vi "ex_getNextGroupTDMS.vi"(8 "error in (no error)":errorcluster, 9 "group index in":u32, 11 "tdms file in":refnum<k34>) -> (0 "error out":errorcluster, 1 "group index out":u32, 2 "group name":string, 3 "tdms file out":refnum<k34>, 4 "is last group?":bool, 5 "max len":i32)   [LabVIEW 2017]
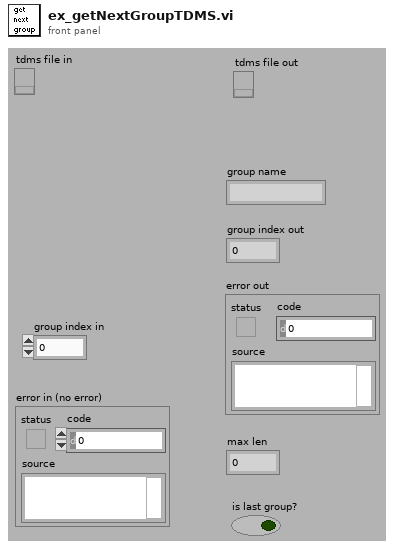
[diagram p1: front panel]
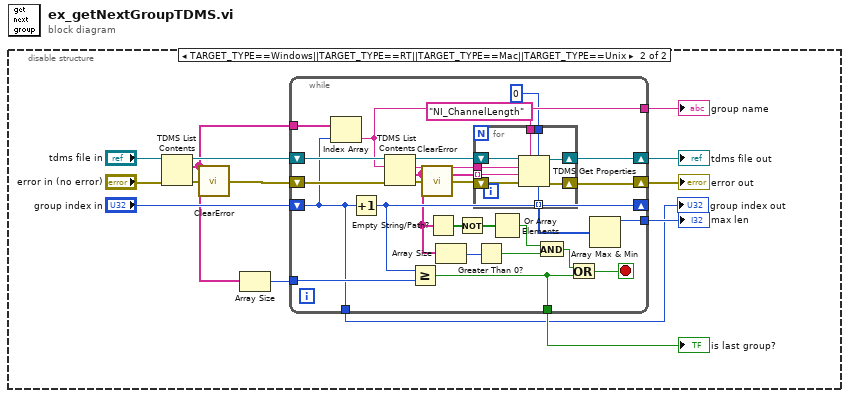
[diagram p0: block diagram]
diagram:
  n1 = disable-structure shown="TARGET_TYPE==Windows||TARGET_TYPE==RT||TARGET_TYPE==Mac||TARGET_TYPE==Unix" {
    frame condition #0 {
    }
    frame condition #1 (active) {
      n2 = TDMS List Contents(4:"error in (no error)", 7:"tdms file in") -> (0:w1:errorcluster, 2:w2:string[], 3:w14:refnum<k34>)  [unwired: 1 in, 1 out]
      n3 = call <vilib>:"ClearError.vi"("error in (no error)"=w1) -> ("error out"=w12:errorcluster)
      n4 = Array Size(array=w2) -> (size(s)=w9:i32)
      n5 = while {
        tunnel: w2 -> [w38]
        tunnel: [w37] -> w6
        shift-right: [w27] -> w5
        shift-left: w12 -> [w40]
        shift-right: [w25] -> w4
        shift-left: w14 -> [w39]
        shift-right: [w17] -> _
        shift-left: "group index in" -> [w18]
        tunnel: w9 -> [w35]
        tunnel: [w20] -> w8
        tunnel: [w19] -> w10
        tunnel: [w18] -> w3
        stop <- w34 stop-if-true
        n6 = Index Array(array=w38, index=w18) -> (element=w37:string)
        n7 = Increment(x=w18) -> (x+1=w17:u32)
        n8 = TDMS List Contents(4:w40, 6:w37, 7:w39) -> (0:w15:errorcluster, 1:w16:string[], 2:w24:string, 3:w26:refnum<k34>)
        n9 = Greater Or Equal?(x=w17, y=w35) -> (x >= y?=w19:bool)
        n10 = call <vilib>:"ClearError.vi"("error in (no error)"=w15) -> ("error out"=w28:errorcluster)
        n11 = Empty String/Path?(string/path=w16) -> (empty?=w33:bool[])
        n12 = Array Size(array=w16) -> (size(s)=w36:i32)
        n13 = Not(x=w33) -> (.not. x?=w32:bool[])
        n14 = for {
          shift-right: [w48] -> w27
          shift-left: w28 -> [w49]
          shift-right: [w46] -> w25
          shift-left: w26 -> [w47]
          tunnel: w24 -> [w45]
          tunnel: w16 -> [w44] mode=indexing
          tunnel: "NI_ChannelLength" -> [w43]
          tunnel: 0 -> [w42]
          tunnel: [w41] -> w21 mode=indexing
          n15 = TDMS Get Properties(5:w42, 7:w43, 8:w49, 9:w44, 10:w45, 11:w47) -> (0:w48:errorcluster, 3:w46:refnum<k34>, 4:w41:i32)  [unwired: 3 out]
        }
        n16 = Greater Than 0?(x=w36) -> (x > 0?=w31:bool)
        n17 = Or Array Elements(Boolean array=w32) -> (logical OR=w29:bool)
        n18 = And(x=w29, y=w31) -> (x .and. y?=w30:bool)
        n19 = Or(x=w30, y=w19) -> (x .or. y?=w34:bool)
        n20 = Array Max & Min(array=w21) -> (max value=w20:i32)  [unwired: 3 out]
      }
      "is last group?" <- w10
      "max len" <- w8
      "group index out" <- w3
      "group name" <- w6
      "error out" <- w5
      "tdms file out" <- w4
    }
  }
